vi "Handle Error.vi"(8 "error in (no error)":errorcluster, 11 "Camera Process in":refnum<class "Camera Process.lvclass">) -> (0 "error out":errorcluster, 2 "stop actor?":bool=TRUE, 3 "Camera Process out":refnum<class "Camera Process.lvclass">)   [LabVIEW 2022 SP3, in "Cam Process.lvlib" / "Camera Process.lvclass"]
doc: "(<B>Filename</B>: Actor Framework.lvlib:Actor.lvclass:Handle Error.vi)\n\nDefines how the actor handles an error that occurred while processing a message.\n\nBy default, this method does nothing except stop the actor. This method also treats error code 43 (coming from <B>error in</B>) as a sign that the actor shut down normally. In this situation, the Handle Error method does not return the error on <B>error out</B>, meaning the actor's caller will not receive it. All other error codes will be returned on <B>error out</B>.\n\nA descendant class may override this method to change this behavior."
uses:
  Camera Process.lvclass
  Camera Process.lvclass/Camera Process.ctl
  XY Stage/Process Actor/Process Framework/Process State Data/Process State Data.lvclass/Process State Data.ctl
  XY Stage/Process Actor/Process Framework/Process State Data/Accessor/Write Proccess Error.vi
  XY Stage/Process Actor/Process Framework/Process State Data/Accessor/Write Busy.vi
  XY Stage/Process Actor/Process Framework/Process State Data/Process State Data.lvclass
  <vilib>/ActorFramework/Actor/Actor.lvclass
  Camera Process Messages/Snap Image Msg/Snap Image Msg.lvclass
  C:/Program Files/National Instruments/LabVIEW 2022/vi.lib/MGI/Monitored Actor/Monitored Actor/Monitored Actor/Monitored Actor.lvclass
  C:/Program Files/National Instruments/LabVIEW 2022/vi.lib/ActorFramework/Actor/Actor.lvclass
  C:/XY Stage/Camera/Camera Process/Camera Process.lvclass
  C:/XY Stage/Camera/Camera API/Camera API.lvclass
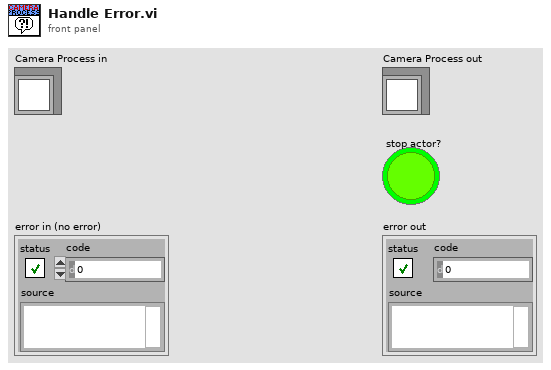
[diagram p1: front panel]
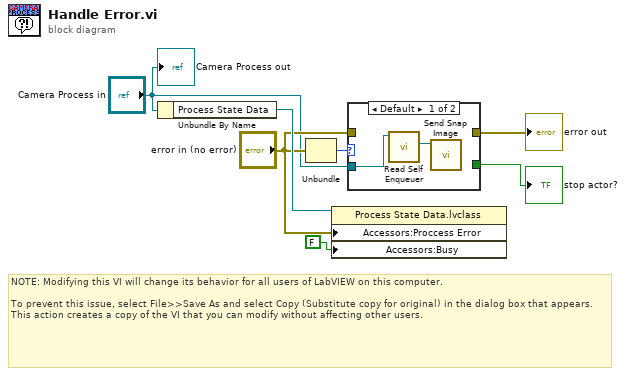
[diagram p0: block diagram]
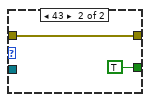
[diagram p2: hidden frame]
diagram:
  # "NOTE: Modifying this VI will change its behavior for all users of LabVIEW on this computer.\n\nTo prevent this issue, select File>>Save As and select Copy (Substitute copy for original) in the dialog box that appears. This action creates a copy of the VI that you can modify without affecting other users."
  n1 = Unbundle By Name("Camera Process in") -> ("Process State Data"=w4:refnum<data-value>)
  n2 = Unbundle("error in (no error)") -> ("code"=w7:i32)  [unwired: 2 out]
  n3 = property class="Process State Data.lvclass"(reference=w4, "Accessors:Proccess Error"="error in (no error)", "Accessors:Busy"=FALSE ("Busy")) -> ()  [unwired: 1 in, 2 out]
  n4 = case shown="Default" w7 {
    tunnel: "error in (no error)" -> [_ w10]
    tunnel: [_ TRUE] -> w6
    tunnel: [_ w10] -> w5
    tunnel: "Camera Process in" -> [w9 _]
    frame Default {
      n5 = call <vilib>:"Read Self Enqueuer.vi"("Actor"=w9) -> ("Self Enqueuer"=w8:refnum<class "Message Enqueuer.lvclass">)  [unwired: 10 in]
      n6 = call "Send Snap Image.vi"("Message Enqueuer"=w8) -> ()  [unwired: 9 in, 2 out]
    }
    frame 43 {
    }
  }
  "error out" <- w5
  "stop actor?" <- w6
  "Camera Process out" <- "Camera Process in"
